vi "Call Subpanel By Reference.vi"() -> ()   [LabVIEW 2018]
doc: "This example demonstrates the easiest method of inserting a VI into a subpanel"
panel:
  out "error out":errorcluster
  out "ADB PID":string
  out "Connectet":bool
  in  "Path":path=path "D:/LABVIEW/SEQUENSER_SNA/Ver_08/BLUETOOTH/ADB-BlueTooth.vi"
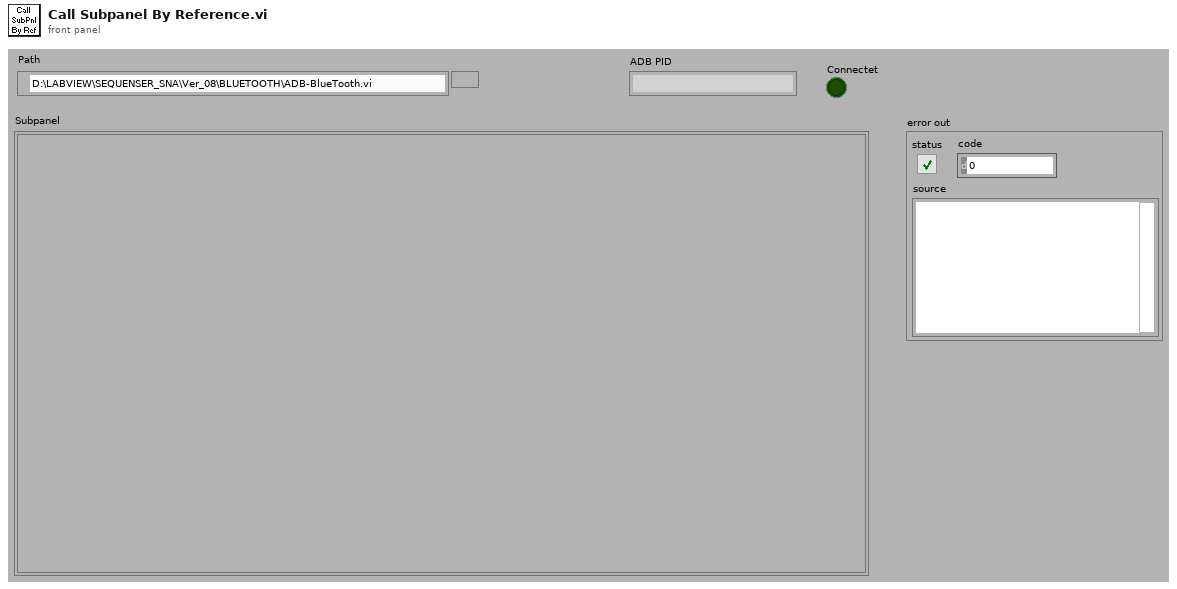
[diagram p1: front panel]
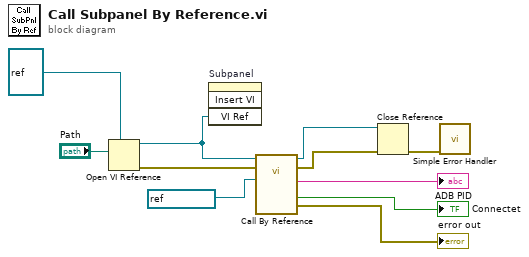
[diagram p0: block diagram]
diagram:
  n1 = Open VI Reference(type specifier VI Refnum (for type only)=refnum<vi> refnum, vi path="Path") -> (vi reference=w2:refnum<vi>, error out=w8:errorcluster)  [unwired: 4 in]
  n2 = invoke on="Subpanel" class="SubPnl" method="Insert VI"("VI Ref"=w2) -> ()  [unwired: 3 in, 4 out]
  n3 = call-by-ref "?"(reference=w2, error in=w8, "COM Port"=refnum<visa-resource-name> "COM18") -> (reference out=w1:refnum<vi>, error out=w5:errorcluster, 0:"error out"=→"error out":errorcluster, "Connectet"=→"Connectet":bool, "ADB PID"=→"ADB PID":string)  [unwired: 7 in, 1 out]
  n4 = Close Reference(reference=w1, error in (no error)=w5) -> (error out=w11:errorcluster)
  n5 = call <vilib>:"Simple Error Handler.vi"("error in (no error)"=w11) -> ()  [unwired: 4 in, 5 out]
